vi "ABB enter motor data.vi"() -> (1 "Efficiency Standard out":u16(ring) items=["IEC", "NEMA"], 2 "Motor Type out":u16(ring) items=["Wound Induction Motor", "Induction Motor", "Synchronous Motor", "Synchronous Generator"], 3 "Entered data":string[][](array[string]), 5 "Efficiency Units out":u16(ring) items=["METRIC", "IMPERIAL", "", "", ""])   [LabVIEW 2017]
uses:
  <vilib>/Analysis/baseanly.llb/Mean (DBL).vi
  ABB global.vi
  <vilib>/Analysis/NI_AALBase.lvlib
panel:
  in  "Efficiency Units":u16(ring) items=["METRIC", "IMPERIAL", "", "", ""]
  in  "Efficiency Standard":u16(ring) items=["IEC 60034", "NEMA", "IEC 61972"]
  in  "Site Ambient Temperature":dbl
  out "Gap":cluster{"Total Gap":dbl, "Air Gap":dbl}
  in  "Air Gap":T1
  in  "Space heater":T2 {"Power (kW)" format="%#_3f"}
  in  "Bearing Data":T3={"Bearing Type DE"=0, "Detector type"=1, "Lubrication"=0, "Primary coolant"=0, "Dim. DE (mm)"=0.0, "Dim. NDE (mm)"=0.0, "No. DE temp. det"=0, "DE  Ohms"=[], "Oil viscosity"=0.0, "Flow rate (l/min)"=0.0, "Hours running"=0.0, "Insulation Test volts (kV)"=0.0, "Bearing insulation DE (MOhm)?"=0.0, "Bearing Insulation NDE (MOhm)"=0.0, "Water Flow Rate"=0.0, "NDE  Ohms"=[], "No. NDE temp. det"=0, "DE Temperature"=0.0, "NDE Temperature"=0.0, "Temperature Rise  Limit"=0.0} {"NDE Temperature" format="%#.2f"; "DE Temperature" format="%#.2f"; "No. NDE temp. det" min=0 max=5; "Bearing Type DE" items=["Sleeve", "Anti-friction"]; "Primary coolant" items=["Oil", "Water", "Natural"]; "Detector type" items=["Thermocouple", "RTD"]; "No. DE temp. det" min=0 max=5; "Lubrication" items=["Oil", "Grease"]}
  in  "Header":T4={"Works order No."="", "Serial No."="", "Type"="", "IC"="", "IM"="", "Specification"="IEC 60034-1 /2004", "Plant"="", "Client"="", "Rated Power"=0.0, "Year of Manufacture"=0, "Mass (kg)"=0.0, "Rated Speed (rpm)"=0.0, "Power Factor"=0.0, "Stator Rated Voltage (V)"=0.0, "Stator Rated Current (A)"=0.0, "Frequency (Hz)"=0.0, "Rotor Rated Voltage (V)"=0.0, "Rotor Rated Current (A)"=0.0, "Duty"=0, "Stator Winding "=0, "Rotor Winding"=0, "IP"=0, "IP10"=0, "Rotation from DE"=0, "Insulation Class"=0, "Number poles"=0} {"IP" items=["0", "1", "2", "3", "4", "5", "6", "7", "8", "9"]; "Rotor Winding" items=["Star", "Delta"]; "Insulation Class" items=["B", "F", "H"]; "Rotation from DE" items=["CW", "CCW", "Bi-Directional"]; "IP10" items=["0", "1", "2", "3", "4", "5", "6", "7", "8", "9"]; "Stator Winding" items=["Star", "Delta"]; "Duty" items=["S1", "S2", "S3"]}
  in  "Shaft":T5
  in  "Brushes & slip rings":T6 {"Brush lifting mech" items=["Yes", "No", "N/A"]; "Brush dimension" items=["25 x 32", "20 x 40"]; "Terminals from DE" items=["Left", "Right", "Top", "Bottom"]}
  in  "Motor Type":u16(ring) items=["Wound Induction Motor", "Induction Motor", "Synchronous Motor", "Synchronous Generator"]
  in  "Exit":bool
  # "Enter Motor data"
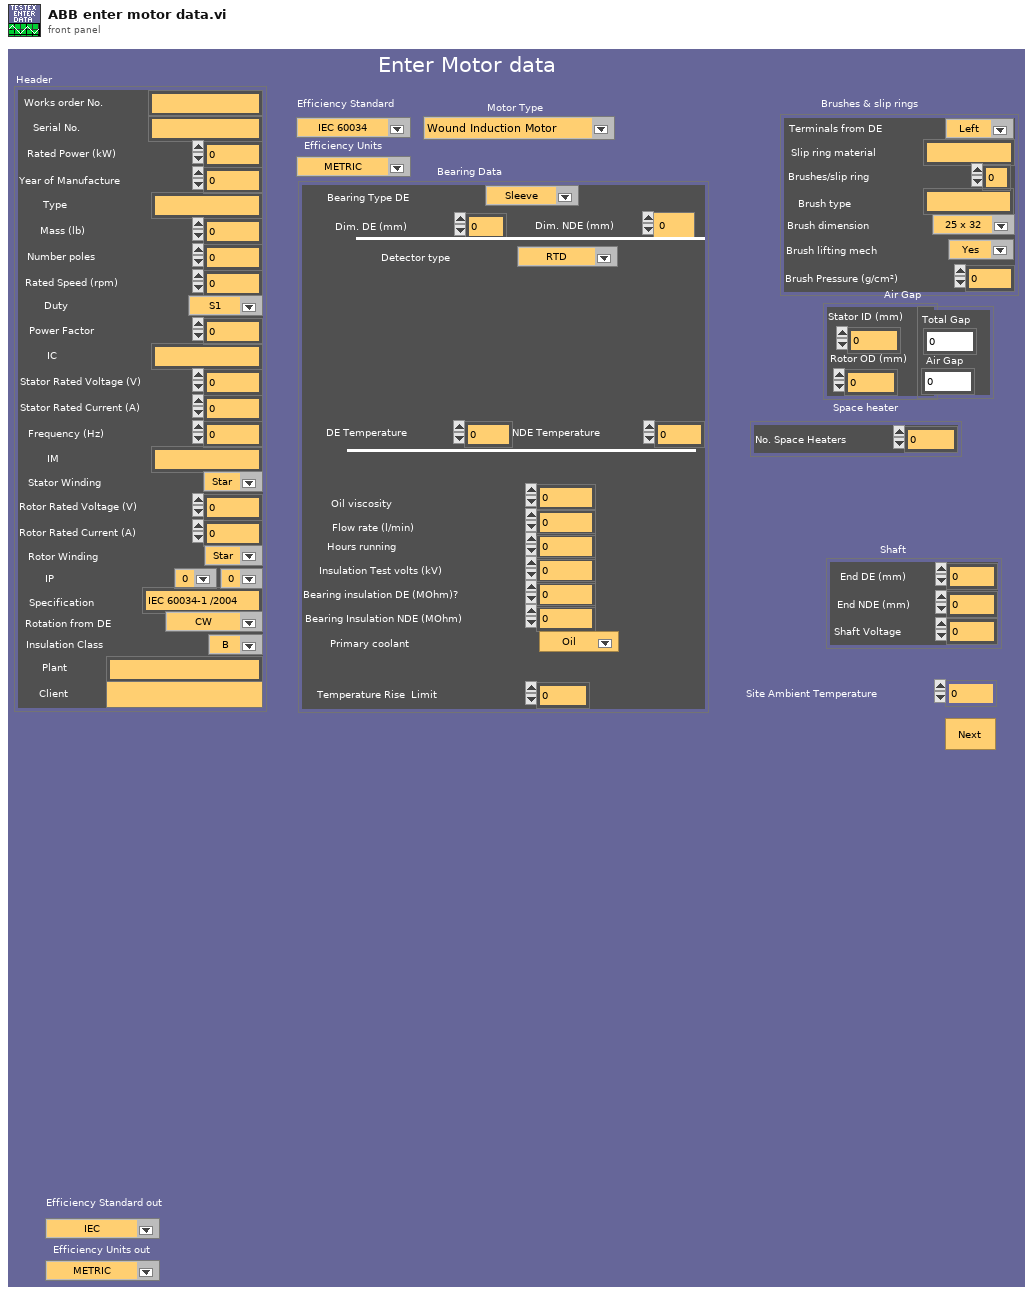
[diagram p1: front panel]
types:
  T1 = cluster{"StatorID (mm)":dbl, "Rotor OD (mm)":dbl}
  T2 = cluster{"No. Space Heaters":i32, "Resistance (Ohms)":dbl[], "Voltage (V)":dbl[], "Power (kW)":dbl[]}
  T3 = cluster{"Bearing Type DE":u16, "Detector type":u16, "Lubrication":u16, "Primary coolant":u16, "Dim. DE (mm)":dbl, "Dim. NDE (mm)":dbl, "No. DE temp. det":i32, "DE  Ohms":dbl[], "Oil viscosity":dbl, "Flow rate (l/min)":dbl, "Hours running":dbl, "Insulation Test volts (kV)":dbl, "Bearing insulation DE (MOhm)?":dbl, "Bearing Insulation NDE (MOhm)":dbl, "Water Flow Rate":dbl, "NDE  Ohms":dbl[], "No. NDE temp. det":i32, "DE Temperature":dbl, "NDE Temperature":dbl, "Temperature Rise  Limit":dbl}
  T4 = cluster{"Works order No.":string, "Serial No.":string, "Type":string, "IC":string, "IM":string, "Specification":string, "Plant":string, "Client":string, "Rated Power":dbl, "Year of Manufacture":i32, "Mass (kg)":dbl, "Rated Speed (rpm)":dbl, "Power Factor":dbl, "Stator Rated Voltage (V)":dbl, "Stator Rated Current (A)":dbl, "Frequency (Hz)":dbl, "Rotor Rated Voltage (V)":dbl, "Rotor Rated Current (A)":dbl, "Duty":u16, "Stator Winding ":u16, "Rotor Winding":u16, "IP":u16, "IP10":u16, "Rotation from DE":u16, "Insulation Class":u16, "Number poles":i32}
  T5 = cluster{" End DE (mm)":dbl, " End NDE (mm)":dbl, " Shaft Voltage":dbl}
  T6 = cluster{"Slip ring material":string, "Brush type":string, "Brushes/slip ring":i32, "Brush Pressure (g/cm²)":dbl, "Terminals from DE":i32, "Brush dimension":i32, "Brush lifting mech":u16}
  T7 = cluster{"String":string, "String":string, "String":string, "String":string, "String":string, "String":string, "String":string, "String":string, "String":string, "String":string}
  T8 = cluster{"String":dbl, "String":dbl, "String":dbl, "String":dbl, "String":dbl, "String":dbl, "String":dbl, "String":dbl, "String":dbl, "String":dbl}
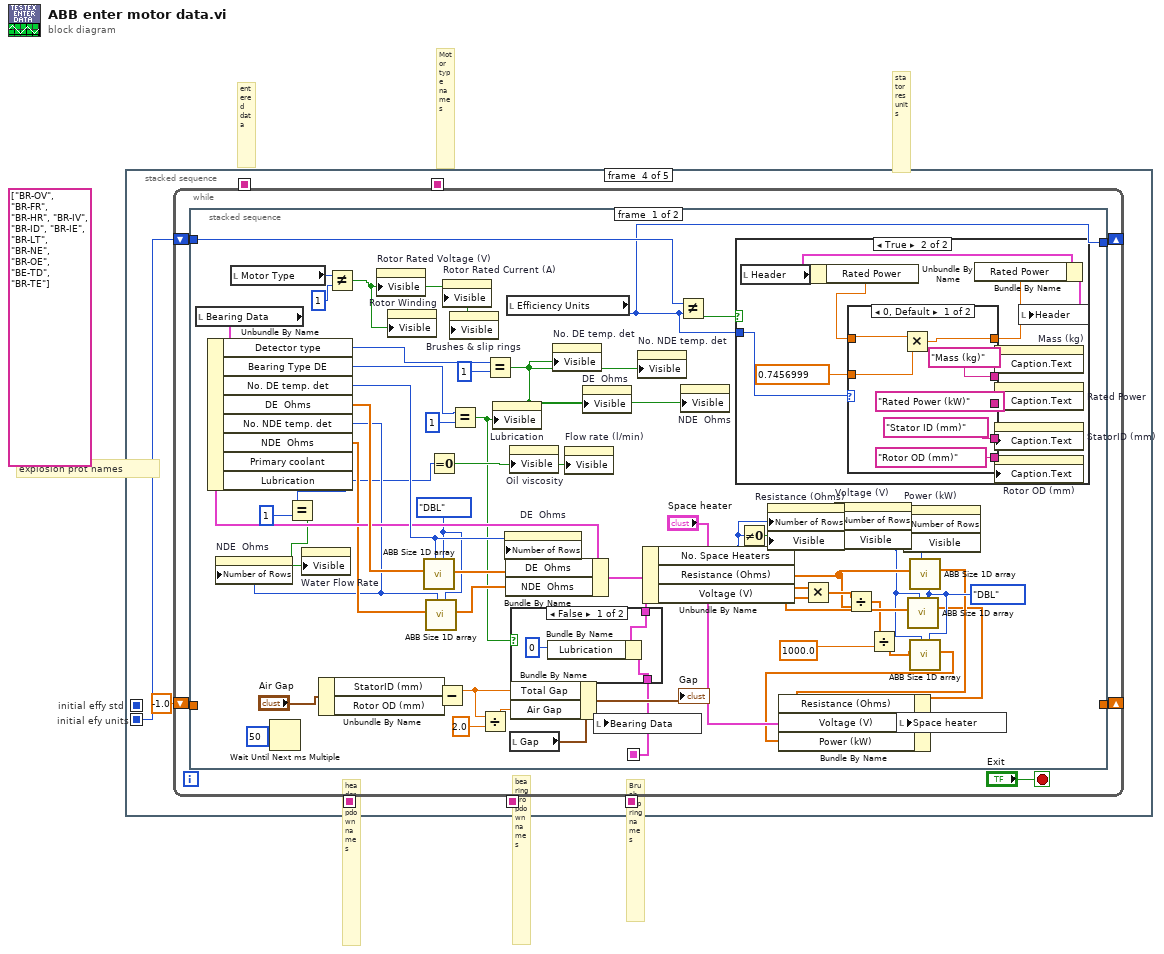
[diagram p0: block diagram]
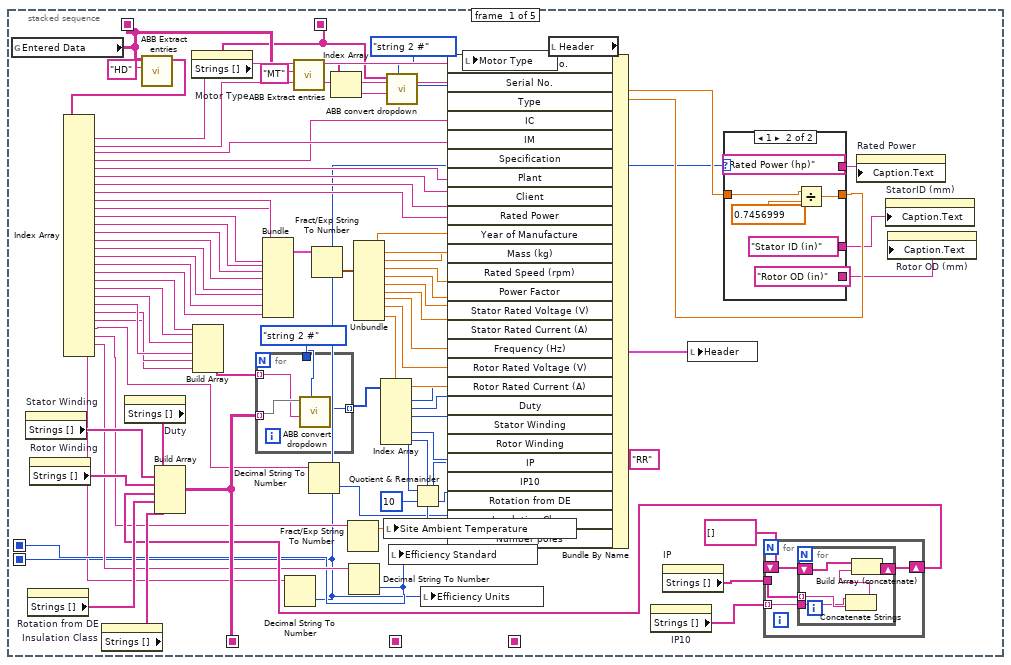
[diagram p2: hidden frame]
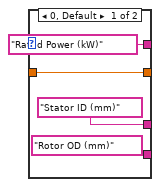
[diagram p3: hidden frame]
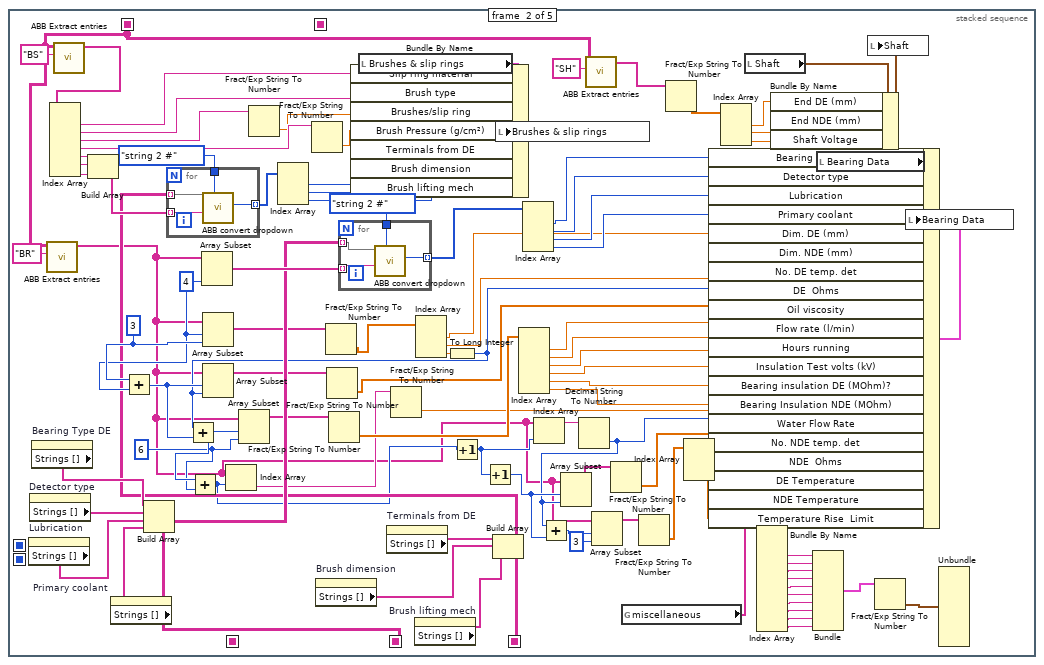
[diagram p4: hidden frame]
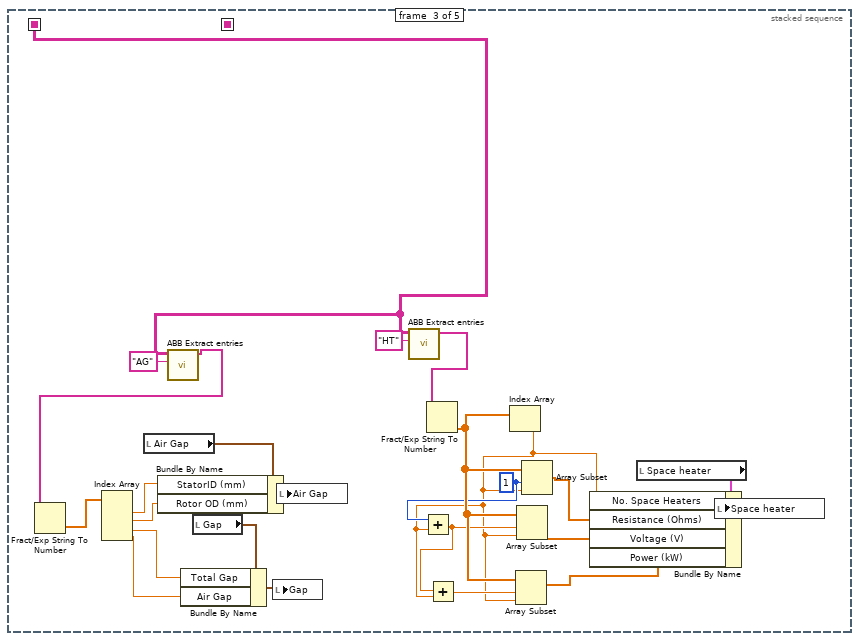
[diagram p5: hidden frame]
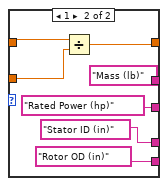
[diagram p7: hidden frame]
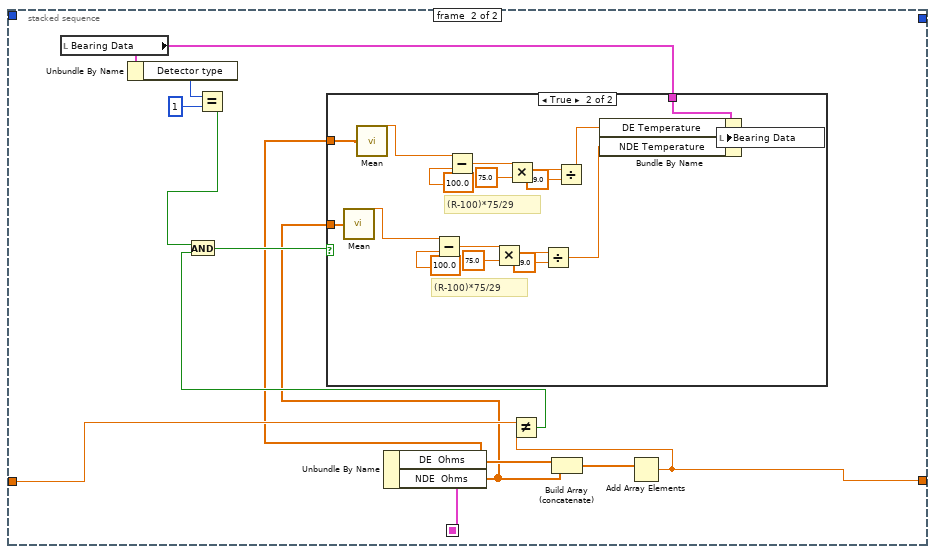
[diagram p9: hidden frame]
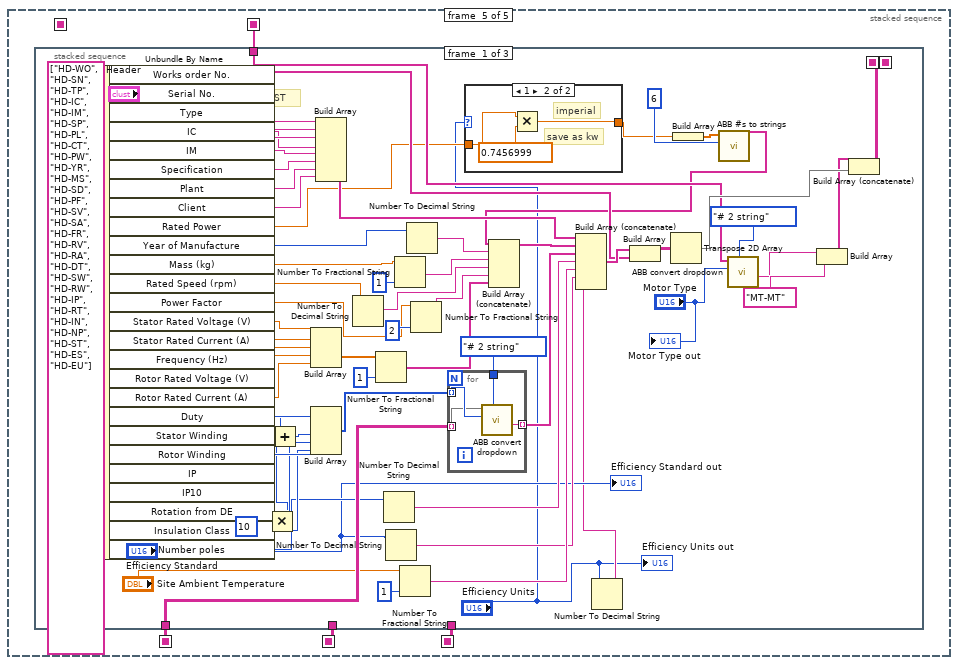
[diagram p11: hidden frame]
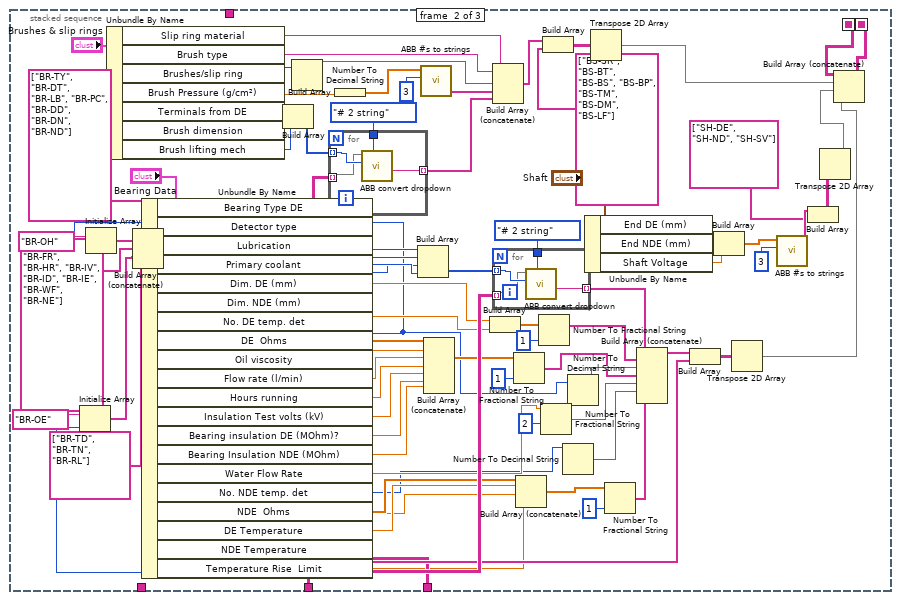
[diagram p13: hidden frame]
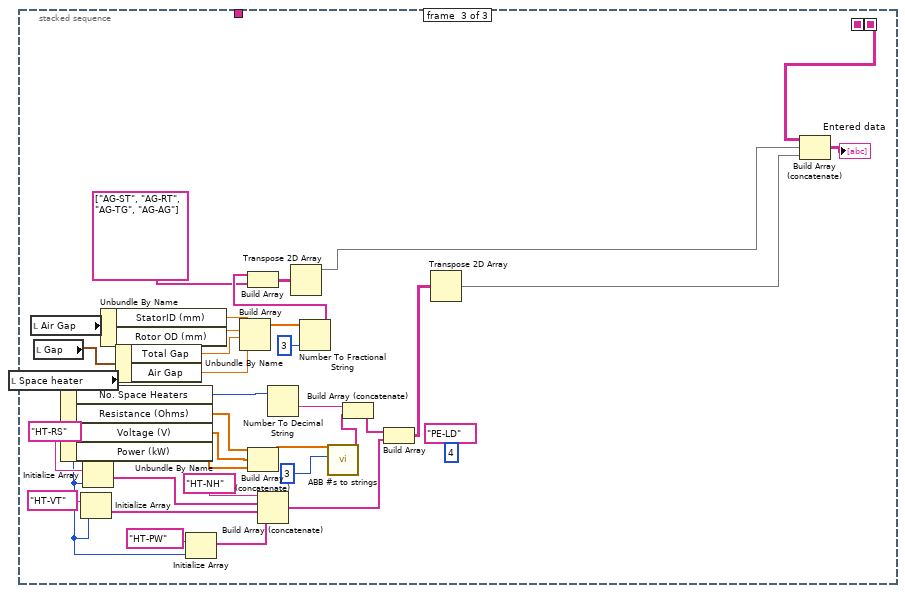
[diagram p14: hidden frame]
diagram:
  (unwired) string[] ["BR-OV", "BR-FR", "BR-HR", "BR-IV", "BR-ID", "BR-IE", "BR-LT", "BR-NE", "BR-OE", "BE-TD", "BR-TE"]
  # "initial efy units"
  # "initial effy std"
  # "Motor type names"
  # "entered data"
  # "explosion prot names"
  # "Brush slipring names"
  # "bearing dropdown names"
  # "header dropdown names"
  # "stator res units"
  n1 = stacked-sequence {
    seq-local: [w41 _ _ _ _] -> [_ _ _ _ w353]
    seq-local: [_ w175 _ _ _] -> [_ _ _ _ w352]
    seq-local: [_ w131 _ _ _] -> [_ _ _ _ w351]
    seq-local: [w23 _ _ _ _] -> [_ w125 w216 _ _]
    seq-local: [w21 _ _ _ _] -> [_ _ _ _ w350]
    seq-local: [w7 _ _ _ _] -> [_ _ _ _ _]
    seq-local: [w1 _ _ _ _] -> [_ _ _ w235 _]
    frame #0 {
      (unwired) "RR" ("Entry ID")
      n2 = global read "ABB global.vi" "Entered Data"() -> (w23:string[][])
      n3 = property on="Stator Winding" class="Ring (strict)"() -> ("Strings []"=w44:string[])  [unwired: 2 in, 2 out]
      n4 = property on="Rotation from DE" class="Ring (strict)"() -> ("Strings []"=w42:string[])  [unwired: 2 in, 2 out]
      n5 = property on="Rotor Winding" class="Ring (strict)"() -> ("Strings []"=w43:string[])  [unwired: 2 in, 2 out]
      n6 = property on="Insulation Class" class="Ring (strict)"() -> ("Strings []"=w46:string[])  [unwired: 2 in, 2 out]
      n7 = property on="Duty" class="Ring (strict)"() -> ("Strings []"=w45:string[])  [unwired: 2 in, 2 out]
      n8 = call "ABB Extract entries.vi"("Entry ID"="HD", "Entry table in"=w23) -> ("Selected Entries"=w25:string[])  [unwired: 9 in]
      n9 = Index Array(array=w25) -> (element #1=w79:string, element #2=w78:string, element #3=w77:string, element #4=w76:string, element #5=w75:string, element #6=w74:string, element #7=w73:string, element #8=w72:string, element #9=w71:string, element #10=w70:string, element #11=w69:string, element #12=w68:string, element #13=w67:string, element #14=w66:string, element #15=w65:string, element #16=w56:string, element #17=w55:string, element #18=w54:string, element #19=w50:string, element #20=w49:string, element #21=w48:string, element #22=w47:string, element #23=w28:string, element #24=w27:string, element #25=w17:string, element #26=w10:string, element #27=w9:string, element #28=w4:string)  [unwired: 28 in]
      n10 = property on="Motor Type" class="Ring (strict)"() -> ("Strings []"=w21:string[])  [unwired: 2 in, 2 out]
      n11 = Build Array(w50, w49, w48, w47, w28, w27) -> (w40:string[])
      n12 = Bundle("String"=w71, "String"=w70, "String"=w69, "String"=w68, "String"=w67, "String"=w66, "String"=w65, "String"=w56, "String"=w55, "String"=w54) -> (w64:T7)  [unwired: 1 in]
      n13 = Decimal String To Number(string=w4) -> (number=w1:i32)  [unwired: 2 in, 1 out]
      n14 = call "ABB Extract entries.vi"("Entry ID"="MT", "Entry table in"=w23) -> ("Selected Entries"=w22:string[])  [unwired: 9 in]
      n15 = Decimal String To Number(string=w17) -> (number=w16:i32)  [unwired: 2 in, 1 out]
      n16 = Fract/Exp String To Number(string=w64) -> (number=w63:T8)  [unwired: 3 in, 1 out]
      n17 = Index Array(array=w22) -> (element=w19:string)  [unwired: 1 in]
      n18 = Fract/Exp String To Number(string=w10) -> (number=w11:dbl)  [unwired: 3 in, 1 out]
      n19 = Decimal String To Number(string=w9) -> (number=w7:i32)  [unwired: 2 in, 1 out]
      n20 = Unbundle(w63) -> ("String"=w6:dbl, "String"=w62:dbl, "String"=w61:dbl, "String"=w60:dbl, "String"=w59:dbl, "String"=w58:dbl, "String"=w57:dbl, "String"=w53:dbl, "String"=w52:dbl, "String"=w51:dbl)
      n21 = local write "Site Ambient Temperature"(w11) -> ()
      n22 = call "ABB convert dropdown.vi"("Mode"=enum16{"# 2 string", "string 2 #"}."string 2 #", "String in"=w19, "Strings"=w21) -> ("#out"=w18:i32)  [unwired: 7 in, 1 out]
      n23 = local write "Efficiency Standard"(w7) -> ()
      n24 = local write "Efficiency Units"(w1) -> ()
      n25 = local write "Motor Type"(w18) -> ()
      n26 = local read "Header"() -> (w81:T4)
      n27 = property on="IP10" class="Ring (strict)"() -> ("Strings []"=w15:string[])  [unwired: 2 in, 2 out]
      n28 = property on="IP" class="Ring (strict)"() -> ("Strings []"=w14:string[])  [unwired: 2 in, 2 out]
      n29 = case shown="1" w1 {
        tunnel: ["Rated Power (kW)" "Rated Power (hp)"] -> w8
        tunnel: w6 -> [w84 w90]
        tunnel: [w84 w89] -> w5
        tunnel: ["Stator ID (mm)" "Stator ID (in)"] -> w3
        tunnel: ["Rotor OD (mm)" "Rotor OD (in)"] -> w2
        frame 0, Default {
        }
        frame 1 {
          n30 = Divide(x=w90, y=0.7456999) -> (x/y=w89:dbl)
        }
      }
      n31 = for {
        tunnel: w15 -> [w94] mode=indexing
        shift-right: [w93] -> w12
        shift-left: string[] [] -> [w92]
        tunnel: w14 -> [w95]
        n32 = for {
          tunnel: w95 -> [w97] mode=indexing
          tunnel: w94 -> [w96]
          shift-right: [w99] -> w93
          shift-left: w92 -> [w98]
          n33 = Concatenate Strings(w96, w97) -> (w100:string)
          n34 = Build Array (concatenate)(w98, w100) -> (w99:string[])
        }
      }
      n35 = Build Array(w45, w44, w43, w12, w42, w46) -> (w41:string[][])
      n36 = for {
        tunnel: w41 -> [w104] mode=indexing
        tunnel: w40 -> [w103] mode=indexing
        tunnel: [w102] -> w39 mode=indexing
        tunnel: enum16{"# 2 string", "string 2 #"}."string 2 #" ("Mode") -> [w101]
        n37 = call "ABB convert dropdown.vi"("Mode"=w101, "String in"=w103, "Strings"=w104) -> ("#out"=w102:i32)  [unwired: 7 in, 1 out]
      }
      n38 = Index Array(array=w39) -> (element #1=w38:i32, element #2=w37:i32, element #3=w36:i32, element #4=w32:i32, element #5=w34:i32, element #6=w33:i32)  [unwired: 6 in]
      n39 = Quotient & Remainder(x=w32, y=10) -> (x-y*floor(x/y)=w29:i32, floor(x/y)=w30:i32)
      n40 = Bundle By Name(cluster=w81, "Works order No."=w79, "Serial No."=w78, "Type"=w77, "IC"=w76, "IM"=w75, "Specification"=w74, "Plant"=w73, "Client"=w72, "Rated Power"=w5, "Year of Manufacture"=w62, "Mass (kg)"=w61, "Rated Speed (rpm)"=w60, "Power Factor"=w59, "Stator Rated Voltage (V)"=w58, "Stator Rated Current (A)"=w57, "Frequency (Hz)"=w53, "Rotor Rated Voltage (V)"=w52, "Rotor Rated Current (A)"=w51, "Duty"=w38, "Stator Winding"=w37, "Rotor Winding"=w36, "IP"=w29, "IP10"=w30, "Rotation from DE"=w34, "Insulation Class"=w33, "Number poles"=w16) -> (w80:T4)
      n41 = local write "Header"(w80) -> ()
      n42 = property on="Rated Power" class="DigNum (strict)"("Caption.Text"=w8) -> ()  [unwired: 2 in, 2 out]
      n43 = property on="StatorID (mm)" class="DigNum (strict)"("Caption.Text"=w3) -> ()  [unwired: 2 in, 2 out]
      n44 = property on="Rotor OD (mm)" class="DigNum (strict)"("Caption.Text"=w2) -> ()  [unwired: 2 in, 2 out]
    }
    frame #1 {
      w151 = 6 ("length")
      w164 = 3 ("length")
      w163 = 4 ("length")
      n45 = property on="Lubrication" class="Ring (strict)"() -> ("Strings []"=w181:string[])  [unwired: 2 in, 2 out]
      n46 = property on="Detector type" class="Ring (strict)"() -> ("Strings []"=w182:string[])  [unwired: 2 in, 2 out]
      n47 = property on="Bearing Type DE" class="Ring (strict)"() -> ("Strings []"=w179:string[])  [unwired: 2 in, 2 out]
      n48 = call "ABB Extract entries.vi"("Entry ID"="BR", "Entry table in"=w125) -> ("Selected Entries"=w116:string[])  [unwired: 9 in]
      n49 = call "ABB Extract entries.vi"("Entry ID"="BS", "Entry table in"=w125) -> ("Selected Entries"=w130:string[])  [unwired: 9 in]
      n50 = Index Array(array=w130) -> (element #1=w145:string, element #2=w144:string, element #3=w143:string, element #4=w142:string, element #5=w135:string, element #6=w134:string, element #7=w133:string)  [unwired: 7 in]
      n51 = Build Array(w135, w134, w133) -> (w132:string[])
      n52 = property on="Primary coolant" class="Ring (strict)"() -> ("Strings []"=w180:string[])  [unwired: 2 in, 2 out]
      n53 = Add(x=w164, y=w163) -> (x+y=w160:i32)
      n54 = Build Array(w179, w182, w181, w180) -> (w175:string[][])
      n55 = Array Subset(array=w116, length=w163) -> (w176:string[])  [unwired: 1 in]
      n56 = Array Subset(array=w116, index=w163, length=w164) -> (w168:string[])
      n57 = Fract/Exp String To Number(string=w143) -> (number=w141:dbl)  [unwired: 3 in, 1 out]
      n58 = Fract/Exp String To Number(string=w142) -> (number=w140:dbl)  [unwired: 3 in, 1 out]
      n59 = property on="Brush dimension" class="Ring (strict)"() -> ("Strings []"=w148:string[])  [unwired: 2 in, 2 out]
      n60 = Fract/Exp String To Number(string=w168) -> (number=w167:dbl[])  [unwired: 3 in, 1 out]
      n61 = for {
        tunnel: w176 -> [w208] mode=indexing
        tunnel: w175 -> [w210] mode=indexing
        tunnel: enum16{"# 2 string", "string 2 #"}."string 2 #" ("Mode") -> [w209]
        tunnel: [w207] -> w173 mode=indexing
        n62 = call "ABB convert dropdown.vi"("Mode"=w209, "String in"=w208, "Strings"=w210) -> ("#out"=w207:i32)  [unwired: 7 in, 1 out]
      }
      n63 = local read "Brushes & slip rings"() -> (w202:T6)
      n64 = property on="Terminals from DE" class="Ring (strict)"() -> ("Strings []"=w149:string[])  [unwired: 2 in, 2 out]
      n65 = property on="Brush lifting mech" class="Ring (strict)"() -> ("Strings []"=w147:string[])  [unwired: 2 in, 2 out]
      n66 = Index Array(array=w167) -> (element #1=w166:dbl, element #2=w165:dbl, element #3=w161:dbl)  [unwired: 3 in]
      n67 = To Long Integer(number=w161) -> (32bit integer=w119:i32)
      n68 = Add(x=w119, y=w160) -> (x+y=w152:i32)
      n69 = Add(x=w152, y=w151) -> (x+y=w124:i32)
      n70 = Array Subset(array=w116, index=w160, length=w119) -> (w162:string[])
      n71 = Index Array(array=w116, index=w124) -> (element=w150:string)
      n72 = Array Subset(array=w116, index=w152, length=w151) -> (w159:string[])
      n73 = Fract/Exp String To Number(string=w162) -> (number=w108:dbl[])  [unwired: 3 in, 1 out]
      n74 = Fract/Exp String To Number(string=w159) -> (number=w158:dbl[])  [unwired: 3 in, 1 out]
      n75 = Fract/Exp String To Number(string=w150) -> (number=w109:dbl)  [unwired: 3 in, 1 out]
      n76 = Increment(x=w124) -> (x+1=w122:i32)
      n77 = Increment(x=w122) -> (x+1=w118:i32)
      n78 = Build Array(w149, w148, w147) -> (w131:string[][])
      n79 = for {
        tunnel: enum16{"# 2 string", "string 2 #"}."string 2 #" ("Mode") -> [w206]
        tunnel: [w205] -> w138 mode=indexing
        tunnel: w132 -> [w204] mode=indexing
        tunnel: w131 -> [w203] mode=indexing
        n80 = call "ABB convert dropdown.vi"("Mode"=w206, "String in"=w204, "Strings"=w203) -> ("#out"=w205:i32)  [unwired: 7 in, 1 out]
      }
      n81 = Index Array(array=w138) -> (element #1=w139:i32, element #2=w137:i32, element #3=w136:i32)  [unwired: 3 in]
      n82 = Bundle By Name(cluster=w202, "Slip ring material"=w145, "Brush type"=w144, "Brushes/slip ring"=w141, "Brush Pressure (g/cm²)"=w140, "Terminals from DE"=w139, "Brush dimension"=w137, "Brush lifting mech"=w136) -> (w201:T6)
      n83 = local write "Brushes & slip rings"(w201) -> ()
      n84 = Index Array(array=w158) -> (element #1=w157:dbl, element #2=w156:dbl, element #3=w155:dbl, element #4=w154:dbl, element #5=w153:dbl, element #6=w106:dbl)  [unwired: 6 in]
      n85 = Index Array(array=w173) -> (element #1=w172:i32, element #2=w171:i32, element #3=w170:i32, element #4=w169:i32)  [unwired: 4 in]
      n86 = Index Array(array=w116, index=w122) -> (element=w123:string)
      n87 = Decimal String To Number(string=w123) -> (number=w117:i32)  [unwired: 2 in, 1 out]
      n88 = Add(x=w117, y=w118) -> (x+y=w115:i32)
      n89 = Array Subset(array=w116, index=w118, length=w117) -> (w121:string[])
      n90 = call "ABB Extract entries.vi"("Entry ID"="SH", "Entry table in"=w125) -> ("Selected Entries"=w127:string[])  [unwired: 9 in]
      n91 = Array Subset(array=w116, index=w115, length=3) -> (w113:string[])
      n92 = Fract/Exp String To Number(string=w121) -> (number=w120:dbl[])  [unwired: 3 in, 1 out]
      n93 = global read "ABB global.vi" "miscellaneous"() -> (w200:string[])
      n94 = Fract/Exp String To Number(string=w113) -> (number=w112:dbl[])  [unwired: 3 in, 1 out]
      n95 = Fract/Exp String To Number(string=w127) -> (number=w187:dbl[])  [unwired: 3 in, 1 out]
      n96 = Index Array(array=w112) -> (element #1=w111:dbl, element #2=w110:dbl, element #3=w107:dbl)  [unwired: 3 in]
      n97 = Index Array(array=w187) -> (element #1=w185:dbl, element #2=w184:dbl, element #3=w105:dbl)  [unwired: 3 in]
      n98 = local read "Shaft"() -> (w186:T5)
      n99 = Index Array(array=w200) -> (element #2=w198:string, element #3=w197:string, element #4=w196:string, element #5=w195:string, element #6=w194:string, element #7=w193:string, element #8=w192:string, element #9=w191:string, element #10=w190:string, element #11=w189:string)  [unwired: 11 in, 1 out]
      n100 = Bundle By Name(cluster=w186, "End DE (mm)"=w185, "End NDE (mm)"=w184, "Shaft Voltage"=w105) -> (w183:T5)
      n101 = Bundle("String"=w198, "String"=w197, "String"=w196, "String"=w195, "String"=w194, "String"=w193, "String"=w192, "String"=w191, "String"=w190, "String"=w189) -> (w188:T7)  [unwired: 1 in]
      n102 = local read "Bearing Data"() -> (w178:T3)
      n103 = Bundle By Name(cluster=w178, "Bearing Type DE"=w172, "Detector type"=w171, "Lubrication"=w170, "Primary coolant"=w169, "Dim. DE (mm)"=w166, "Dim. NDE (mm)"=w165, "No. DE temp. det"=w119, "DE  Ohms"=w108, "Oil viscosity"=w157, "Flow rate (l/min)"=w156, "Hours running"=w155, "Insulation Test volts (kV)"=w154, "Bearing insulation DE (MOhm)?"=w153, "Bearing Insulation NDE (MOhm)"=w106, "Water Flow Rate"=w109, "No. NDE temp. det"=w117, "NDE  Ohms"=w120, "DE Temperature"=w111, "NDE Temperature"=w110, "Temperature Rise  Limit"=w107) -> (w177:T3)
      n104 = local write "Shaft"(w183) -> ()
      n105 = Fract/Exp String To Number(string=w188) -> (number=w199:T8)  [unwired: 3 in, 1 out]
      n106 = local write "Bearing Data"(w177) -> ()
      n107 = Unbundle(w199) -> ()  [unwired: 10 out]
    }
    frame #2 {
      w228 = 1 ("index")
      n108 = local read "Air Gap"() -> (w234:T1)
      n109 = call "ABB Extract entries.vi"("Entry ID"="AG", "Entry table in"=w216) -> ("Selected Entries"=w215:string[])  [unwired: 9 in]
      n110 = Fract/Exp String To Number(string=w215) -> (number=w233:dbl[])  [unwired: 3 in, 1 out]
      n111 = Index Array(array=w233) -> (element #1=w232:dbl, element #2=w231:dbl, element #3=w212:dbl, element #4=w211:dbl)  [unwired: 4 in]
      n112 = Bundle By Name(cluster=w234, "StatorID (mm)"=w232, "Rotor OD (mm)"=w231) -> (w230:T1)
      n113 = local read "Gap"() -> (w214:cluster{"Total Gap":dbl, "Air Gap":dbl})
      n114 = Bundle By Name(cluster=w214, "Total Gap"=w212, "Air Gap"=w211) -> (w213:cluster{"Total Gap":dbl, "Air Gap":dbl})
      n115 = local write "Gap"(w213) -> ()
      n116 = local write "Air Gap"(w230) -> ()
      n117 = call "ABB Extract entries.vi"("Entry ID"="HT", "Entry table in"=w216) -> ("Selected Entries"=w218:string[])  [unwired: 9 in]
      n118 = Fract/Exp String To Number(string=w218) -> (number=w229:dbl[])  [unwired: 3 in, 1 out]
      n119 = Index Array(array=w229) -> (element=w224:dbl)  [unwired: 1 in]
      n120 = Add(x=w228, y=w224) -> (x+y=w227:dbl)
      n121 = Add(x=w227, y=w224) -> (x+y=w226:dbl)
      n122 = Array Subset(array=w229, index=w226, length=w224) -> (w220:dbl[])
      n123 = Array Subset(array=w229, index=w227, length=w224) -> (w221:dbl[])
      n124 = Array Subset(array=w229, index=w228, length=w224) -> (w222:dbl[])
      n125 = local read "Space heater"() -> (w225:T2)
      n126 = Bundle By Name(cluster=w225, "No. Space Heaters"=w224, "Resistance (Ohms)"=w222, "Voltage (V)"=w221, "Power (kW)"=w220) -> (w223:T2)
      n127 = local write "Space heater"(w223) -> ()
    }
    frame #3 {
      n128 = while {
        shift-right: [w239] -> _
        shift-left: -1.0 ("Average bearing") -> [w240]
        shift-right: [w238] -> _
        shift-left: w235 -> [w237]
        stop <- "Exit" stop-if-true
        n129 = stacked-sequence {
          seq-local: [w245 _] -> [_ w330]
          tunnel: w240 -> [_ w331]
          tunnel: [_ w329] -> w239
          tunnel: [w242 _] -> w238
          tunnel: w237 -> [w244 _]
          frame #0 {
            w272 = enum16{"Integer", "DBL", "STRING", "BOOLEAN"}."DBL" ("Type")
            w262 = enum16{"Integer", "DBL", "STRING", "BOOLEAN"}."DBL" ("Type")
            n130 = local read "Bearing Data"() -> (w284:T3)
            n131 = Unbundle By Name(w284) -> ("Detector type"=w289:u16, "Bearing Type DE"=w248:u16, "No. DE temp. det"=w286:i32, "DE  Ohms"=w285:dbl[], "No. NDE temp. det"=w260:i32, "NDE  Ohms"=w263:dbl[], "Primary coolant"=w253:u16, "Lubrication"=w250:u16)
            n132 = property on="NDE  Ohms" class="Arr (strict)"("Number of Rows"=w260) -> ()  [unwired: 2 in, 2 out]
            n133 = local read "Motor Type"() -> (w291:u16)
            n134 = Wait Until Next ms Multiple(millisecond multiple=u32 50) -> ()  [unwired: 1 out]
            n135 = Equal?(x=w253, y=u16 1) -> (x = y?=w251:bool)
            n136 = property on="Water Flow Rate" class="DigNum (strict)"("Visible"=w251) -> ()  [unwired: 2 in, 2 out]
            n137 = Unbundle By Name("Air Gap") -> ("StatorID (mm)"=w281:dbl, "Rotor OD (mm)"=w280:dbl)
            n138 = Not Equal?(x=w291, y=u16 1) -> (x != y?=w264:bool)
            n139 = property on="Rotor Rated Voltage (V)" class="DigNum (strict)"("Visible"=w264) -> ()  [unwired: 2 in, 2 out]
            n140 = property on="Rotor Winding" class="Ring (strict)"("Visible"=w264) -> ()  [unwired: 2 in, 2 out]
            n141 = call "ABB Size 1D array.vi"("Type"=w262, "Size"=w286, "DBL Array In"=w285) -> ("DBL Array out"=w283:dbl[])  [unwired: 5 in, 3 out]
            n142 = call "ABB Size 1D array.vi"("Type"=w262, "Size"=w260, "DBL Array In"=w263) -> ("DBL Array out"=w261:dbl[])  [unwired: 5 in, 3 out]
            n143 = Equal To 0?(x=w250) -> (x = 0?=w249:bool)
            n144 = Subtract(x=w281, y=w280) -> (x-y=w256:dbl)
            n145 = property on="Rotor Rated Current (A)" class="DigNum (strict)"("Visible"=w264) -> ()  [unwired: 2 in, 2 out]
            n146 = property on="Brushes & slip rings" class="Clust (strict)"("Visible"=w264) -> ()  [unwired: 2 in, 2 out]
            n147 = Equal?(x=w248, y=u16 1) -> (x = y?=w247:bool)
            n148 = Divide(x=w256, y=2.0) -> (x/y=w254:dbl)
            n149 = Equal?(x=w289, y=u16 1) -> (x = y?=w259:bool)
            n150 = property on="Lubrication" class="Ring (strict)"("Visible"=w247) -> ()  [unwired: 2 in, 2 out]
            n151 = property on="DE  Ohms" class="Arr (strict)"("Number of Rows"=w286) -> ()  [unwired: 2 in, 2 out]
            n152 = Bundle By Name(cluster=w284, "DE  Ohms"=w283, "NDE  Ohms"=w261) -> (w246:T3)
            n153 = local read "Efficiency Units"() -> (w242:u16)
            n154 = property on="Oil viscosity" class="DigNum (strict)"("Visible"=w249) -> ()  [unwired: 2 in, 2 out]
            n155 = local read "Gap"() -> (w258:cluster{"Total Gap":dbl, "Air Gap":dbl})
            n156 = case shown="False" w247 {
              tunnel: w246 -> [w318 w319]
              tunnel: [w317 w319] -> w245
              frame False {
                n157 = Bundle By Name(cluster=w318, "Lubrication"=0) -> (w317:T3)
              }
              frame True {
              }
            }
            n158 = Bundle By Name(cluster=w258, "Total Gap"=w256, "Air Gap"=w254) -> (→"Gap":cluster{"Total Gap":dbl, "Air Gap":dbl})
            n159 = property on="No. DE temp. det" class="DigNum (strict)"("Visible"=w259) -> ()  [unwired: 2 in, 2 out]
            n160 = property on="Flow rate (l/min)" class="DigNum (strict)"("Visible"=w249) -> ()  [unwired: 2 in, 2 out]
            n161 = property on="DE  Ohms" class="Arr (strict)"("Visible"=w259) -> ()  [unwired: 2 in, 2 out]
            n162 = local write "Bearing Data"(w245) -> ()
            n163 = property on="No. NDE temp. det" class="DigNum (strict)"("Visible"=w259) -> ()  [unwired: 2 in, 2 out]
            n164 = Unbundle By Name("Space heater") -> ("No. Space Heaters"=w273:i32, "Resistance (Ohms)"=w276:dbl[], "Voltage (V)"=w275:dbl[])
            n165 = Not Equal?(x=w244, y=w242) -> (x != y?=w243:bool)
            n166 = property on="NDE  Ohms" class="Arr (strict)"("Visible"=w259) -> ()  [unwired: 2 in, 2 out]
            n167 = case shown="True" w243 {
              tunnel: w242 -> [_ w301]
              frame False {
              }
              frame True {
                n168 = local read "Header"() -> (w298:T4)
                n169 = Unbundle By Name(w298) -> ("Rated Power"=w299:dbl)
                n170 = case shown="0, Default" w301 {
                  tunnel: ["Rated Power (kW)" "Rated Power (hp)"] -> w300
                  tunnel: w299 -> [w307 w314]
                  tunnel: [w306 w313] -> w297
                  tunnel: 0.7456999 -> [w305 w312]
                  tunnel: ["Mass (kg)" "Mass (lb)"] -> w294
                  tunnel: ["Stator ID (mm)" "Stator ID (in)"] -> w293
                  tunnel: ["Rotor OD (mm)" "Rotor OD (in)"] -> w292
                  frame 0, Default {
                    n171 = Multiply(x=w307, y=w305) -> (x*y=w306:dbl)
                  }
                  frame 1 {
                    n172 = Divide(x=w314, y=w312) -> (x/y=w313:dbl)
                  }
                }
                n173 = Bundle By Name(cluster=w298, "Rated Power"=w297) -> (w296:T4)
                n174 = property on="Mass (kg)" class="DigNum (strict)"("Caption.Text"=w294) -> ()  [unwired: 2 in, 2 out]
                n175 = property on="Rated Power" class="DigNum (strict)"("Caption.Text"=w300) -> ()  [unwired: 2 in, 2 out]
                n176 = property on="StatorID (mm)" class="DigNum (strict)"("Caption.Text"=w293) -> ()  [unwired: 2 in, 2 out]
                n177 = property on="Rotor OD (mm)" class="DigNum (strict)"("Caption.Text"=w292) -> ()  [unwired: 2 in, 2 out]
                n178 = local write "Header"(w296) -> ()
              }
            }
            n179 = Not Equal To 0?(x=w273) -> (x != 0?=w278:bool)
            n180 = property on="Resistance (Ohms)" class="Arr (strict)"("Number of Rows"=w273, "Visible"=w278) -> ()  [unwired: 2 in, 2 out]
            n181 = Multiply(x=w275, y=w275) -> (x*y=w277:dbl[])
            n182 = property on="Voltage (V)" class="Arr (strict)"("Number of Rows"=w273, "Visible"=w278) -> ()  [unwired: 2 in, 2 out]
            n183 = Divide(x=w277, y=w276) -> (x/y=w274:dbl[])
            n184 = Divide(x=w274, y=1000.0 ("Average bearing")) -> (x/y=w266:dbl[])
            n185 = property on="Power (kW)" class="Arr (strict)"("Number of Rows"=w273, "Visible"=w278) -> ()  [unwired: 2 in, 2 out]
            n186 = call "ABB Size 1D array.vi"("Type"=w272, "Size"=w273, "DBL Array In"=w275) -> ("DBL Array out"=w269:dbl[])  [unwired: 5 in, 3 out]
            n187 = call "ABB Size 1D array.vi"("Type"=w272, "Size"=w273, "DBL Array In"=w276) -> ("DBL Array out"=w270:dbl[])  [unwired: 5 in, 3 out]
            n188 = call "ABB Size 1D array.vi"("Type"=w272, "Size"=w273, "DBL Array In"=w266) -> ("DBL Array out"=w268:dbl[])  [unwired: 5 in, 3 out]
            n189 = Bundle By Name(cluster="Space heater", "Resistance (Ohms)"=w270, "Voltage (V)"=w269, "Power (kW)"=w268) -> (w267:T2)
            n190 = local write "Space heater"(w267) -> ()
          }
          frame #1 {
            n191 = local read "Bearing Data"() -> (w326:T3)
            n192 = Unbundle By Name(w326) -> ("Detector type"=w325:u16)
            n193 = Equal?(x=w325, y=u16 1) -> (x = y?=w323:bool)
            n194 = Unbundle By Name(w330) -> ("DE  Ohms"=w322:dbl[], "NDE  Ohms"=w321:dbl[])
            n195 = Build Array (concatenate)(w322, w321) -> (w320:dbl[])
            n196 = Add Array Elements(numeric array=w320) -> (sum=w329:dbl)
            n197 = Not Equal?(x=w331, y=w329) -> (x != y?=w328:bool)
            n198 = And(x=w323, y=w328) -> (x .and. y?=w327:bool)
            n199 = case shown="True" w327 {
              tunnel: w322 -> [_ w344]
              tunnel: w321 -> [_ w336]
              tunnel: w326 -> [_ w335]
              frame False {
              }
              frame True {
                # "(R-100)*75/29"
                # "(R-100)*75/29"
                n200 = call-poly <vilib>:"Mean.vi"("X"=w336) -> ("mean"=w342:dbl)  [unwired: 1 out]
                n201 = call-poly <vilib>:"Mean.vi"("X"=w344) -> ("mean"=w343:dbl)  [unwired: 1 out]
                n202 = Subtract(x=w342, y=100.0) -> (x-y=w340:dbl)
                n203 = Subtract(x=w343, y=100.0) -> (x-y=w346:dbl)
                n204 = Multiply(x=w340, y=75.0) -> (x*y=w338:dbl)
                n205 = Multiply(x=w346, y=75.0) -> (x*y=w348:dbl)
                n206 = Divide(x=w338, y=29.0) -> (x/y=w332:dbl)
                n207 = Divide(x=w348, y=29.0) -> (x/y=w334:dbl)
                n208 = Bundle By Name(cluster=w335, "DE Temperature"=w334, "NDE Temperature"=w332) -> (w333:T3)
                n209 = local write "Bearing Data"(w333) -> ()
              }
            }
          }
        }
      }
    }
    frame #4 {
      n210 = stacked-sequence {
        seq-local: [w389 _ _] -> [_ w464 _]
        seq-local: [_ w460 _] -> [_ _ w538]
        tunnel: w353 -> [w399 _ _]
        tunnel: w352 -> [_ w499 _]
        tunnel: w351 -> [_ w443 _]
        tunnel: w350 -> [w386 _ _]
        frame #0 {
          # "#HD-ST"
          n211 = Unbundle By Name("Header") -> ("Works order No."=w418:string, "Serial No."=w417:string, "Type"=w416:string, "IC"=w415:string, "IM"=w414:string, "Specification"=w413:string, "Plant"=w412:string, "Client"=w411:string, "Rated Power"=w374:dbl, "Year of Manufacture"=w370:i32, "Mass (kg)"=w367:dbl, "Rated Speed (rpm)"=w364:dbl, "Power Factor"=w359:dbl, "Stator Rated Voltage (V)"=w410:dbl, "Stator Rated Current (A)"=w409:dbl, "Frequency (Hz)"=w377:dbl, "Rotor Rated Voltage (V)"=w408:dbl, "Rotor Rated Current (A)"=w407:dbl, "Duty"=w406:u16, "Stator Winding"=w405:u16, "Rotor Winding"=w404:u16, "IP"=w394:u16, "IP10"=w397:u16, "Rotation from DE"=w403:u16, "Insulation Class"=w402:u16, "Number poles"=w382:i32)
          n212 = Multiply(x=w397, y=u16 10) -> (x*y=w393:u16)
          n213 = Add(x=w394, y=w393) -> (x+y=w395:u16)
          n214 = Build Array(w410, w409, w377, w408, w407) -> (w362:dbl[])
          n215 = Build Array(w406, w405, w404, w395, w403, w402) -> (w398:u16[])
          n216 = Build Array(w418, w417, w416, w415, w414, w413, w412, w411) -> (w420:string[])
          n217 = Number To Decimal String(number=w364) -> (decimal integer string=w363:string)  [unwired: 1 in]
          n218 = Number To Fractional String(number=w362, precision (6)=i16 1) -> (F-format string=w360:string[])  [unwired: 2 in]
          n219 = Number To Decimal String(number=w382) -> (decimal integer string=w381:string)  [unwired: 1 in]
          n220 = Number To Decimal String(number="Efficiency Standard") -> (decimal integer string=w376:string)  [unwired: 1 in]
          n221 = Number To Fractional String(number=w367, precision (6)=i16 1) -> (F-format string=w368:string)  [unwired: 2 in]
          n222 = Number To Fractional String(number="Site Ambient Temperature", precision (6)=i16 1) -> (F-format string=w378:string)  [unwired: 2 in]
          n223 = Number To Decimal String(number=w370) -> (decimal integer string=w372:string)  [unwired: 1 in]
          n224 = Number To Fractional String(number=w359, precision (6)=i16 2) -> (F-format string=w365:string)  [unwired: 2 in]
          n225 = for {
            tunnel: w399 -> [w427] mode=indexing
            tunnel: w398 -> [w428] mode=indexing
            tunnel: enum16{"# 2 string", "string 2 #"}."# 2 string" ("Mode") -> [w429]
            tunnel: [w426] -> w400 mode=indexing
            n226 = call "ABB convert dropdown.vi"("Mode"=w429, "# in"=w428, "Strings"=w427) -> ("String out"=w426:string)  [unwired: 7 in, 1 out]
          }
          n227 = case shown="1" "Efficiency Units" {
            tunnel: w374 -> [w422 w425]
            tunnel: [w422 w424] -> w356
            frame 0, Default {
              # "metric"
            }
            frame 1 {
              # "save as kw"
              # "imperial"
              n228 = Multiply(x=w425, y=0.7456999) -> (x*y=w424:dbl)
            }
          }
          n229 = Number To Decimal String(number="Efficiency Units") -> (decimal integer string=w373:string)  [unwired: 1 in]
          n230 = Build Array(w356) -> (w355:dbl[])
          n231 = call "ABB #s to strings.vi"("Precision"=i16 6 ("precision (6)"), "Numbers in"=w355) -> ("Strings out"=w357:string[])  [unwired: 9 in]
          n232 = Build Array (concatenate)(w357, w372, w368, w363, w365, w360) -> (w371:string[])
          n233 = Build Array (concatenate)(w420, w371, w400, w381, w378, w376, w373) -> (w419:string[])
          n234 = Build Array(w419, string[] ["HD-WO", "HD-SN", "HD-TP", "HD-IC", "HD-IM", "HD-SP", "HD-PL", "HD-CT", "HD-PW", "HD-YR", "HD-MS", "HD-SD", "HD-PF", "HD-SV", "HD-SA", "HD-FR", "HD-RV", "HD-RA", "HD-DT", "HD-SW", "HD-RW", "HD-IP", "HD-RT", "HD-IN", "HD-NP", "HD-ST", "HD-ES", "HD-EU"]) -> (w392:string[][])
          n235 = Transpose 2D Array(2D array=w392) -> (transposed array=w390:string[][])
          n236 = call "ABB convert dropdown.vi"("Mode"=enum16{"# 2 string", "string 2 #"}."# 2 string", "# in"="Motor Type", "Strings"=w386) -> ("String out"=w385:string)  [unwired: 7 in, 1 out]
          n237 = Build Array(w385, "MT-MT") -> (w384:string[])
          n238 = Build Array (concatenate)(w384, w390) -> (w389:string[][])
          "Motor Type out" <- "Motor Type"
          "Efficiency Standard out" <- "Efficiency Standard"
          "Efficiency Units out" <- "Efficiency Units"
        }
        frame #1 {
          n239 = Unbundle By Name("Brushes & slip rings") -> ("Slip ring material"=w479:string, "Brush type"=w478:string, "Brushes/slip ring"=w457:i32, "Brush Pressure (g/cm²)"=w481:dbl, "Terminals from DE"=w485:i32, "Brush dimension"=w484:i32, "Brush lifting mech"=w483:u16)
          n240 = Unbundle By Name("Bearing Data") -> ("Bearing Type DE"=w503:u16, "Detector type"=w502:u16, "Lubrication"=w433:u16, "Primary coolant"=w501:u16, "Dim. DE (mm)"=w438:dbl, "Dim. NDE (mm)"=w437:dbl, "No. DE temp. det"=w434:i32, "DE  Ohms"=w497:dbl[], "Oil viscosity"=w496:dbl, "Flow rate (l/min)"=w495:dbl, "Hours running"=w494:dbl, "Insulation Test volts (kV)"=w493:dbl, "Bearing insulation DE (MOhm)?"=w492:dbl, "Bearing Insulation NDE (MOhm)"=w491:dbl, "Water Flow Rate"=w445:dbl, "No. NDE temp. det"=w441:i32, "NDE  Ohms"=w455:dbl[], "DE Temperature"=w454:dbl, "NDE Temperature"=w453:dbl, "Temperature Rise  Limit"=w442:dbl)
          n241 = Initialize Array("BR-OE", w441) -> (w449:string[])
          n242 = Initialize Array("BR-OH", w434) -> (w470:string[])
          n243 = Build Array (concatenate)(string[] ["BR-TY", "BR-DT", "BR-LB", "BR-PC", "BR-DD", "BR-DN", "BR-ND"], w470, string[] ["BR-OV", "BR-FR", "BR-HR", "BR-IV", "BR-ID", "BR-IE", "BR-WF", "BR-NE"], w449, string[] ["BR-TD", "BR-TN", "BR-RL"]) -> (w467:string[])
          n244 = Build Array(w485, w484, w483) -> (w482:i32[])
          n245 = Number To Decimal String(number=w457) -> (decimal integer string=w456:string)  [unwired: 1 in]
          n246 = for {
            tunnel: w482 -> [w514] mode=indexing
            tunnel: w443 -> [w513] mode=indexing
            tunnel: enum16{"# 2 string", "string 2 #"}."# 2 string" ("Mode") -> [w512]
            tunnel: [w511] -> w476 mode=indexing
            n247 = call "ABB convert dropdown.vi"("Mode"=w512, "# in"=w514, "Strings"=w513) -> ("String out"=w511:string)  [unwired: 7 in, 1 out]
          }
          n248 = Build Array(w481) -> (w480:dbl[])
          n249 = Build Array(w503, w502, w433, w501) -> (w500:u16[])
          n250 = call "ABB #s to strings.vi"("Precision"=i16 3 ("precision (6)"), "Numbers in"=w480) -> ("Strings out"=w477:string[])  [unwired: 9 in]
          n251 = Build Array (concatenate)(w497, w496, w495, w494, w493, w492, w491) -> (w490:dbl[])
          n252 = Build Array(w438, w437) -> (w436:dbl[])
          n253 = Build Array (concatenate)(w479, w478, w456, w477, w476) -> (w475:string[])
          n254 = for {
            tunnel: w500 -> [w518] mode=indexing
            tunnel: w499 -> [w517] mode=indexing
            tunnel: enum16{"# 2 string", "string 2 #"}."# 2 string" ("Mode") -> [w516]
            tunnel: [w515] -> w488 mode=indexing
            n255 = call "ABB convert dropdown.vi"("Mode"=w516, "# in"=w518, "Strings"=w517) -> ("String out"=w515:string)  [unwired: 7 in, 1 out]
          }
          n256 = Number To Fractional String(number=w490, precision (6)=i16 1) -> (F-format string=w431:string[])  [unwired: 2 in]
          n257 = Build Array (concatenate)(w455, w454, w453, w442) -> (w452:dbl[])
          n258 = Number To Fractional String(number=w436, precision (6)=i16 1) -> (F-format string=w435:string[])  [unwired: 2 in]
          n259 = Number To Fractional String(number=w445, precision (6)=i16 2) -> (F-format string=w446:string)  [unwired: 2 in]
          n260 = Build Array(w475, string[] ["BS-SR", "BS-BT", "BS-BS", "BS-BP", "BS-TM", "BS-DM", "BS-LF"]) -> (w474:string[][])
          n261 = Number To Decimal String(number=w441) -> (decimal integer string=w440:string)  [unwired: 1 in]
          n262 = Number To Decimal String(number=w434) -> (decimal integer string=w432:string)  [unwired: 1 in]
          n263 = Unbundle By Name("Shaft") -> ("End DE (mm)"=w508:dbl, "End NDE (mm)"=w507:dbl, "Shaft Voltage"=w430:dbl)
          n264 = Transpose 2D Array(2D array=w474) -> (transposed array=w463:string[][])
          n265 = Number To Fractional String(number=w452, precision (6)=i16 1) -> (F-format string=w447:string[])  [unwired: 2 in]
          n266 = Build Array (concatenate)(w488, w435, w432, w431, w446, w440, w447) -> (w487:string[])
          n267 = Build Array(w487, w467) -> (w468:string[][])
          n268 = Build Array(w508, w507, w430) -> (w505:dbl[])
          n269 = Transpose 2D Array(2D array=w468) -> (transposed array=w461:string[][])
          n270 = call "ABB #s to strings.vi"("Precision"=i16 3 ("precision (6)"), "Numbers in"=w505) -> ("Strings out"=w506:string[])  [unwired: 9 in]
          n271 = Build Array(w506, string[] ["SH-DE", "SH-ND", "SH-SV"]) -> (w465:string[][])
          n272 = Transpose 2D Array(2D array=w465) -> (transposed array=w462:string[][])
          n273 = Build Array (concatenate)(w464, w463, w462, w461) -> (w460:string[][])
        }
        frame #2 {
          (unwired) 4 ("dimension size")
          (unwired) "PE-LD"
          n274 = local read "Space heater"() -> (w547:T2)
          n275 = local read "Air Gap"() -> (w552:T1)
          n276 = local read "Gap"() -> (w521:cluster{"Total Gap":dbl, "Air Gap":dbl})
          n277 = Unbundle By Name(w547) -> ("No. Space Heaters"=w526:i32, "Resistance (Ohms)"=w546:dbl[], "Voltage (V)"=w545:dbl[], "Power (kW)"=w544:dbl[])
          n278 = Initialize Array("HT-VT", w526) -> (w532:string[])
          n279 = Initialize Array("HT-RS", w526) -> (w533:string[])
          n280 = Unbundle By Name(w552) -> ("StatorID (mm)"=w551:dbl, "Rotor OD (mm)"=w550:dbl)
          n281 = Unbundle By Name(w521) -> ("Total Gap"=w520:dbl, "Air Gap"=w519:dbl)
          n282 = Initialize Array("HT-PW", w526) -> (w531:string[])
          n283 = Build Array(w551, w550, w520, w519) -> (w549:dbl[])
          n284 = Build Array (concatenate)(w546, w545, w544) -> (w524:dbl[])
          n285 = Build Array (concatenate)("HT-NH", w533, w532, w531) -> (w529:string[])
          n286 = Number To Decimal String(number=w526) -> (decimal integer string=w525:string)  [unwired: 1 in]
          n287 = Number To Fractional String(number=w549, precision (6)=i16 3) -> (F-format string=w543:string[])  [unwired: 2 in]
          n288 = Build Array(w543, string[] ["AG-ST", "AG-RT", "AG-TG", "AG-AG"]) -> (w541:string[][])
          n289 = Transpose 2D Array(2D array=w541) -> (transposed array=w540:string[][])
          n290 = call "ABB #s to strings.vi"("Precision"=i16 3 ("precision (6)"), "Numbers in"=w524) -> ("Strings out"=w522:string[])  [unwired: 9 in]
          n291 = Build Array (concatenate)(w525, w522) -> (w523:string[])
          n292 = Build Array(w523, w529) -> (w539:string[][])
          n293 = Transpose 2D Array(2D array=w539) -> (transposed array=w537:string[][])
          n294 = Build Array (concatenate)(w538, w540, w537) -> (→"Entered data":string[][])
        }
      }
    }
  }
